vi "Global 1.vi"() -> ()   [LabVIEW 2022 SP3]
panel:
  out "SLM indicator":bool
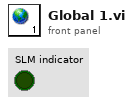
[diagram p1: front panel]
diagram:
